vi "GEOM_TAMP2LL.vi"(9 "AMPROIcoords":T1, 10 "Amplifier":T2={"number"=0, "type"=0, "rotated"=0, "fliped"=0, "FPAcoord"={"xstart"=1, "ystart"=1}, "Physical_size"={"columns"=0, "rows"=0}, "predata"={"columns"=0, "rows"=0}, "postdata"={"columns"=0, "rows"=0}, "Req ROIs"=[], "Corr ROI"=[], "Detnumber"=0, "ampID"="", "discard"=0} {"fliped" items=["none", "horizontal", "vertical"]; "type" items=["LL", "LR", "UL", "UR"]}) -> (1 "DETROICoords":T1)   [LabVIEW 2016]
uses:
  GEOM_Amplifier.ctl
  GEOM_AmpType.ctl
  GEOM_ROI.ctl
  GEOM_Coords.ctl
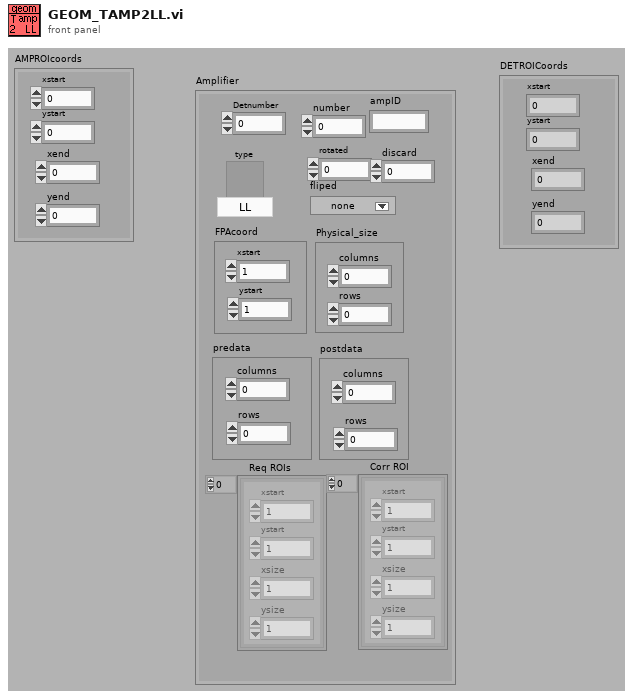
[diagram p1: front panel]
types:
  T1 = cluster{"xstart":i32, "ystart":i32, "xend":i32, "yend":i32}
  T2 = typedef "GEOM_Amplifier.ctl" = cluster{"number":i32, "type":T3, "rotated":i16, "fliped":u16, "FPAcoord":cluster{"xstart":i32, "ystart":i32}, "Physical_size":cluster{"columns":i32, "rows":i32}, "predata":cluster{"columns":i32, "rows":i32}, "postdata":cluster{"columns":i32, "rows":i32}, "Req ROIs":T4, "Corr ROI":T4, "Detnumber":i32, "ampID":string, "discard":i32}
  T3 = typedef "GEOM_AmpType.ctl" = u16
  T4 = typedef "GEOM_ROI.ctl" = T5[]
  T5 = typedef "GEOM_Coords.ctl" = cluster{"xstart":u32, "ystart":u32, "xsize":u32, "ysize":u32}
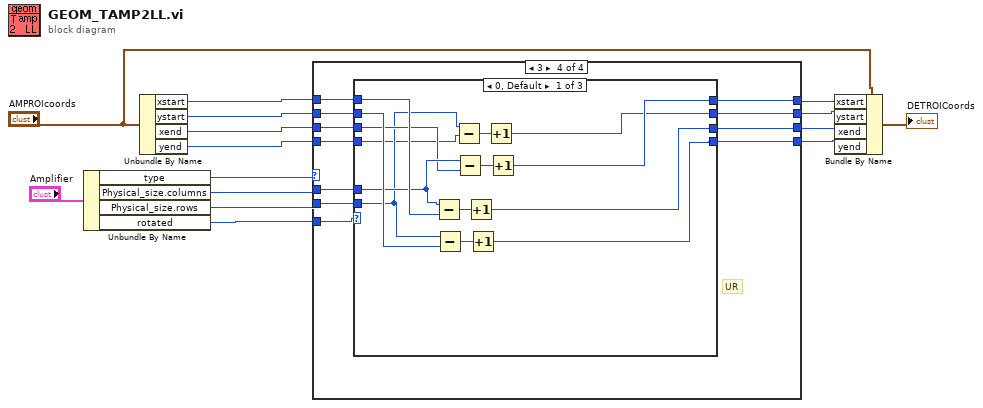
[diagram p0: block diagram]
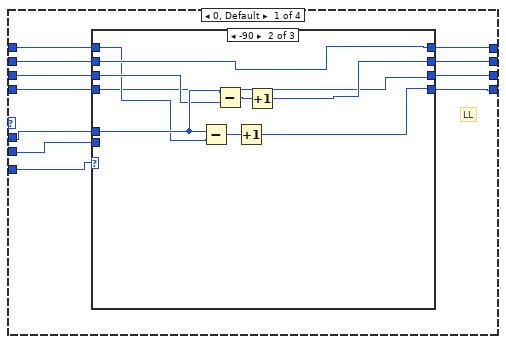
[diagram p2: hidden frame]
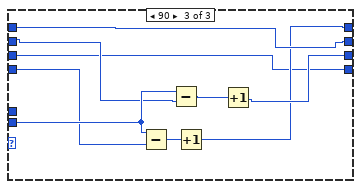
[diagram p4: hidden frame]
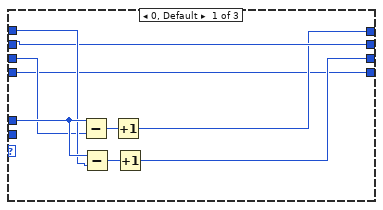
[diagram p6: hidden frame]
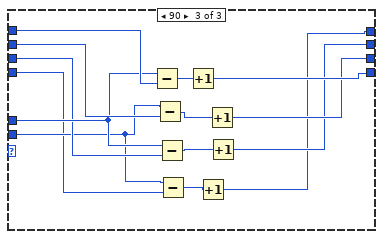
[diagram p7: hidden frame]
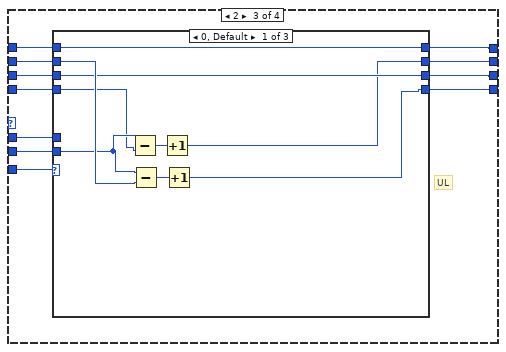
[diagram p8: hidden frame]
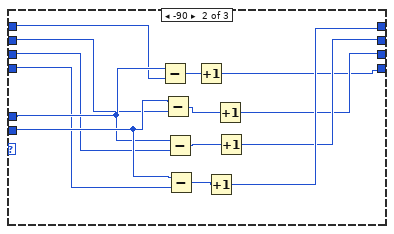
[diagram p9: hidden frame]
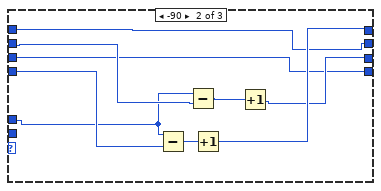
[diagram p11: hidden frame]
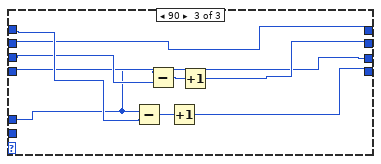
[diagram p12: hidden frame]
diagram:
  n1 = Unbundle By Name("Amplifier") -> ("type"=w14:T3, "Physical_size.columns"=w13:i32, "Physical_size.rows"=w12:i32, "rotated"=w1:i16)
  n2 = Unbundle By Name("AMPROIcoords") -> ("xstart"=w8:i32, "ystart"=w9:i32, "xend"=w10:i32, "yend"=w11:i32)
  n3 = case shown="3" w14 {
    tunnel: w13 -> [w17 w57 w87 w134]
    tunnel: w12 -> [w16 w49 w95 w130]
    tunnel: w11 -> [w19 w53 w97 w135]
    tunnel: w10 -> [w21 w58 w89 w133]
    tunnel: w9 -> [w23 w51 w96 w131]
    tunnel: w8 -> [w25 w59 w91 w132]
    tunnel: [w24 w56 w90 w128] -> w5
    tunnel: [w22 w50 w94 w127] -> w4
    tunnel: [w20 w55 w88 w129] -> w3
    tunnel: [w18 w52 w93 w126] -> w2
    tunnel: w1 -> [w26 w54 w92 w125]
    frame 0, Default {
      # "LL"
      n4 = case shown="-90" w26 {
        tunnel: w25 -> [w30 w33 w45]
        tunnel: [w30 w35 w41] -> w24
        tunnel: w23 -> [w29 w35 w44]
        tunnel: [w29 w32 w45] -> w22
        tunnel: w21 -> [w28 w34 w40]
        tunnel: [w28 w31 w43] -> w20
        tunnel: w19 -> [w27 w31 w42]
        tunnel: [w27 w36 w40] -> w18
        tunnel: w17 -> [_ w38 _]
        tunnel: w16 -> [_ _ w47]
        frame 0, Default {
        }
        frame -90 {
          n5 = Subtract(x=w38, y=w33) -> (x-y=w39:i32)
          n6 = Subtract(x=w38, y=w34) -> (x-y=w37:i32)
          n7 = Increment(x=w39) -> (x+1=w36:i32)
          n8 = Increment(x=w37) -> (x+1=w32:i32)
        }
        frame 90 {
          n9 = Subtract(x=w47, y=w42) -> (x-y=w48:i32)
          n10 = Subtract(x=w47, y=w44) -> (x-y=w46:i32)
          n11 = Increment(x=w48) -> (x+1=w41:i32)
          n12 = Increment(x=w46) -> (x+1=w43:i32)
        }
      }
    }
    frame 1 {
      # "LR"
      n13 = case shown="-90" w54 {
        tunnel: w59 -> [w65 w72 w82]
        tunnel: w58 -> [w62 w70 w77]
        tunnel: w57 -> [w66 _ w78]
        tunnel: [w61 w71 w73] -> w56
        tunnel: [w64 w69 w79] -> w55
        tunnel: w53 -> [w60 w69 w74]
        tunnel: [w60 w70 w81] -> w52
        tunnel: w51 -> [w63 w71 w80]
        tunnel: [w63 w72 w76] -> w50
        tunnel: w49 -> [_ _ w75]
        frame 0, Default {
          n14 = Subtract(x=w66, y=w62) -> (x-y=w68:i32)
          n15 = Subtract(x=w66, y=w65) -> (x-y=w67:i32)
          n16 = Increment(x=w68) -> (x+1=w61:i32)
          n17 = Increment(x=w67) -> (x+1=w64:i32)
        }
        frame -90 {
        }
        frame 90 {
          n18 = Subtract(x=w78, y=w82) -> (x-y=w86:i32)
          n19 = Subtract(x=w75, y=w80) -> (x-y=w84:i32)
          n20 = Subtract(x=w78, y=w77) -> (x-y=w83:i32)
          n21 = Subtract(x=w75, y=w74) -> (x-y=w85:i32)
          n22 = Increment(x=w86) -> (x+1=w81:i32)
          n23 = Increment(x=w85) -> (x+1=w73:i32)
          n24 = Increment(x=w84) -> (x+1=w79:i32)
          n25 = Increment(x=w83) -> (x+1=w76:i32)
        }
      }
    }
    frame 2 {
      # "UL"
      n26 = case shown="0, Default" w92 {
        tunnel: w97 -> [w99 w114 w121]
        tunnel: w96 -> [w103 w112 w123]
        tunnel: w95 -> [w100 w116 _]
        tunnel: [w98 w109 w124] -> w94
        tunnel: [w102 w107 w122] -> w93
        tunnel: w91 -> [w104 w111 w124]
        tunnel: [w104 w110 w123] -> w90
        tunnel: w89 -> [w101 w113 w122]
        tunnel: [w101 w108 w121] -> w88
        tunnel: w87 -> [_ w115 _]
        frame 0, Default {
          n27 = Subtract(x=w100, y=w99) -> (x-y=w106:i32)
          n28 = Subtract(x=w100, y=w103) -> (x-y=w105:i32)
          n29 = Increment(x=w106) -> (x+1=w98:i32)
          n30 = Increment(x=w105) -> (x+1=w102:i32)
        }
        frame -90 {
          n31 = Subtract(x=w115, y=w111) -> (x-y=w120:i32)
          n32 = Subtract(x=w116, y=w112) -> (x-y=w118:i32)
          n33 = Subtract(x=w115, y=w113) -> (x-y=w117:i32)
          n34 = Subtract(x=w116, y=w114) -> (x-y=w119:i32)
          n35 = Increment(x=w120) -> (x+1=w107:i32)
          n36 = Increment(x=w119) -> (x+1=w110:i32)
          n37 = Increment(x=w118) -> (x+1=w108:i32)
          n38 = Increment(x=w117) -> (x+1=w109:i32)
        }
        frame 90 {
        }
      }
    }
    frame 3 {
      # "UR"
      n39 = case shown="0, Default" w125 {
        tunnel: w135 -> [w137 w155 w160]
        tunnel: w134 -> [w141 w154 w159]
        tunnel: w133 -> [w140 w150 w161]
        tunnel: w132 -> [w145 w152 w163]
        tunnel: w131 -> [w143 w156 w162]
        tunnel: w130 -> [w138 _ _]
        tunnel: [w144 w151 w160] -> w129
        tunnel: [w139 w153 w162] -> w128
        tunnel: [w136 w152 w164] -> w127
        tunnel: [w142 w150 w165] -> w126
        frame 0, Default {
          n40 = Subtract(x=w141, y=w145) -> (x-y=w149:i32)
          n41 = Subtract(x=w138, y=w143) -> (x-y=w148:i32)
          n42 = Subtract(x=w138, y=w137) -> (x-y=w146:i32)
          n43 = Subtract(x=w141, y=w140) -> (x-y=w147:i32)
          n44 = Increment(x=w149) -> (x+1=w144:i32)
          n45 = Increment(x=w148) -> (x+1=w142:i32)
          n46 = Increment(x=w146) -> (x+1=w136:i32)
          n47 = Increment(x=w147) -> (x+1=w139:i32)
        }
        frame -90 {
          n48 = Subtract(x=w154, y=w155) -> (x-y=w158:i32)
          n49 = Subtract(x=w154, y=w156) -> (x-y=w157:i32)
          n50 = Increment(x=w158) -> (x+1=w153:i32)
          n51 = Increment(x=w157) -> (x+1=w151:i32)
        }
        frame 90 {
          n52 = Subtract(x=w159, y=w163) -> (x-y=w167:i32)
          n53 = Subtract(x=w159, y=w161) -> (x-y=w166:i32)
          n54 = Increment(x=w167) -> (x+1=w165:i32)
          n55 = Increment(x=w166) -> (x+1=w164:i32)
        }
      }
    }
  }
  n56 = Bundle By Name(cluster="AMPROIcoords", "xstart"=w5, "ystart"=w4, "xend"=w3, "yend"=w2) -> (→"DETROICoords":T1)
